vi "Keithley2200series_2.vi"() -> ()   [LabVIEW 2010]
uses:
  <vilib>/Utility/error.llb/whitespace.ctl
  C:/Users/rad/Desktop/Keithley 2200 Series Power Supplies Ver 1.2 (LV2009)/Keithley 2200 Series/Keithley 2200 Series.lvlib
panel:
  in  "ИС":string="5962-9683901MPA"
  in  "№ ИС":string
  out "SEE1 Count 2":dbl
  out "SEE1 Count":dbl
  in  "SEE th 2":dbl
  in  "SEE th 1":dbl
  in  "+ИП2":bool
  out "MEAS 2":string
  in  "Cml set 2":dbl
  in  "Function(0:Voltage) 3":u16(ring) items=["Voltage", "Current"]
  in  "Out set 2":dbl
  in  "VISA resource name 2":refnum<visa-resource-name>
  in  "Cml set":dbl
  in  "Function(0:Voltage) 2":u16(ring) items=["Voltage", "Current"]
  in  "Out set":dbl
  in  "Файл записи замеров":path
  out "MEAS":string
  in  "VISA resource name":refnum<visa-resource-name>
  in  "stop":bool
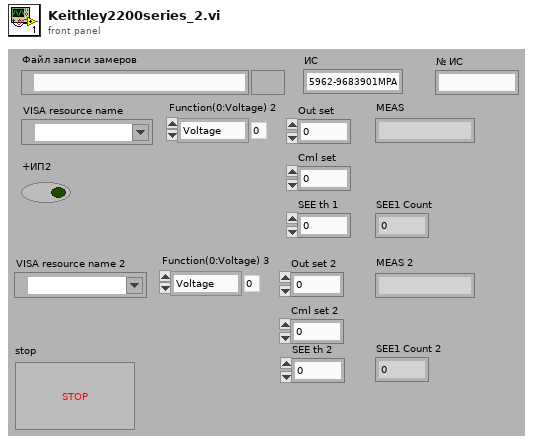
[diagram p1: front panel]
types:
  T1 = typedef "whitespace.ctl" = u16
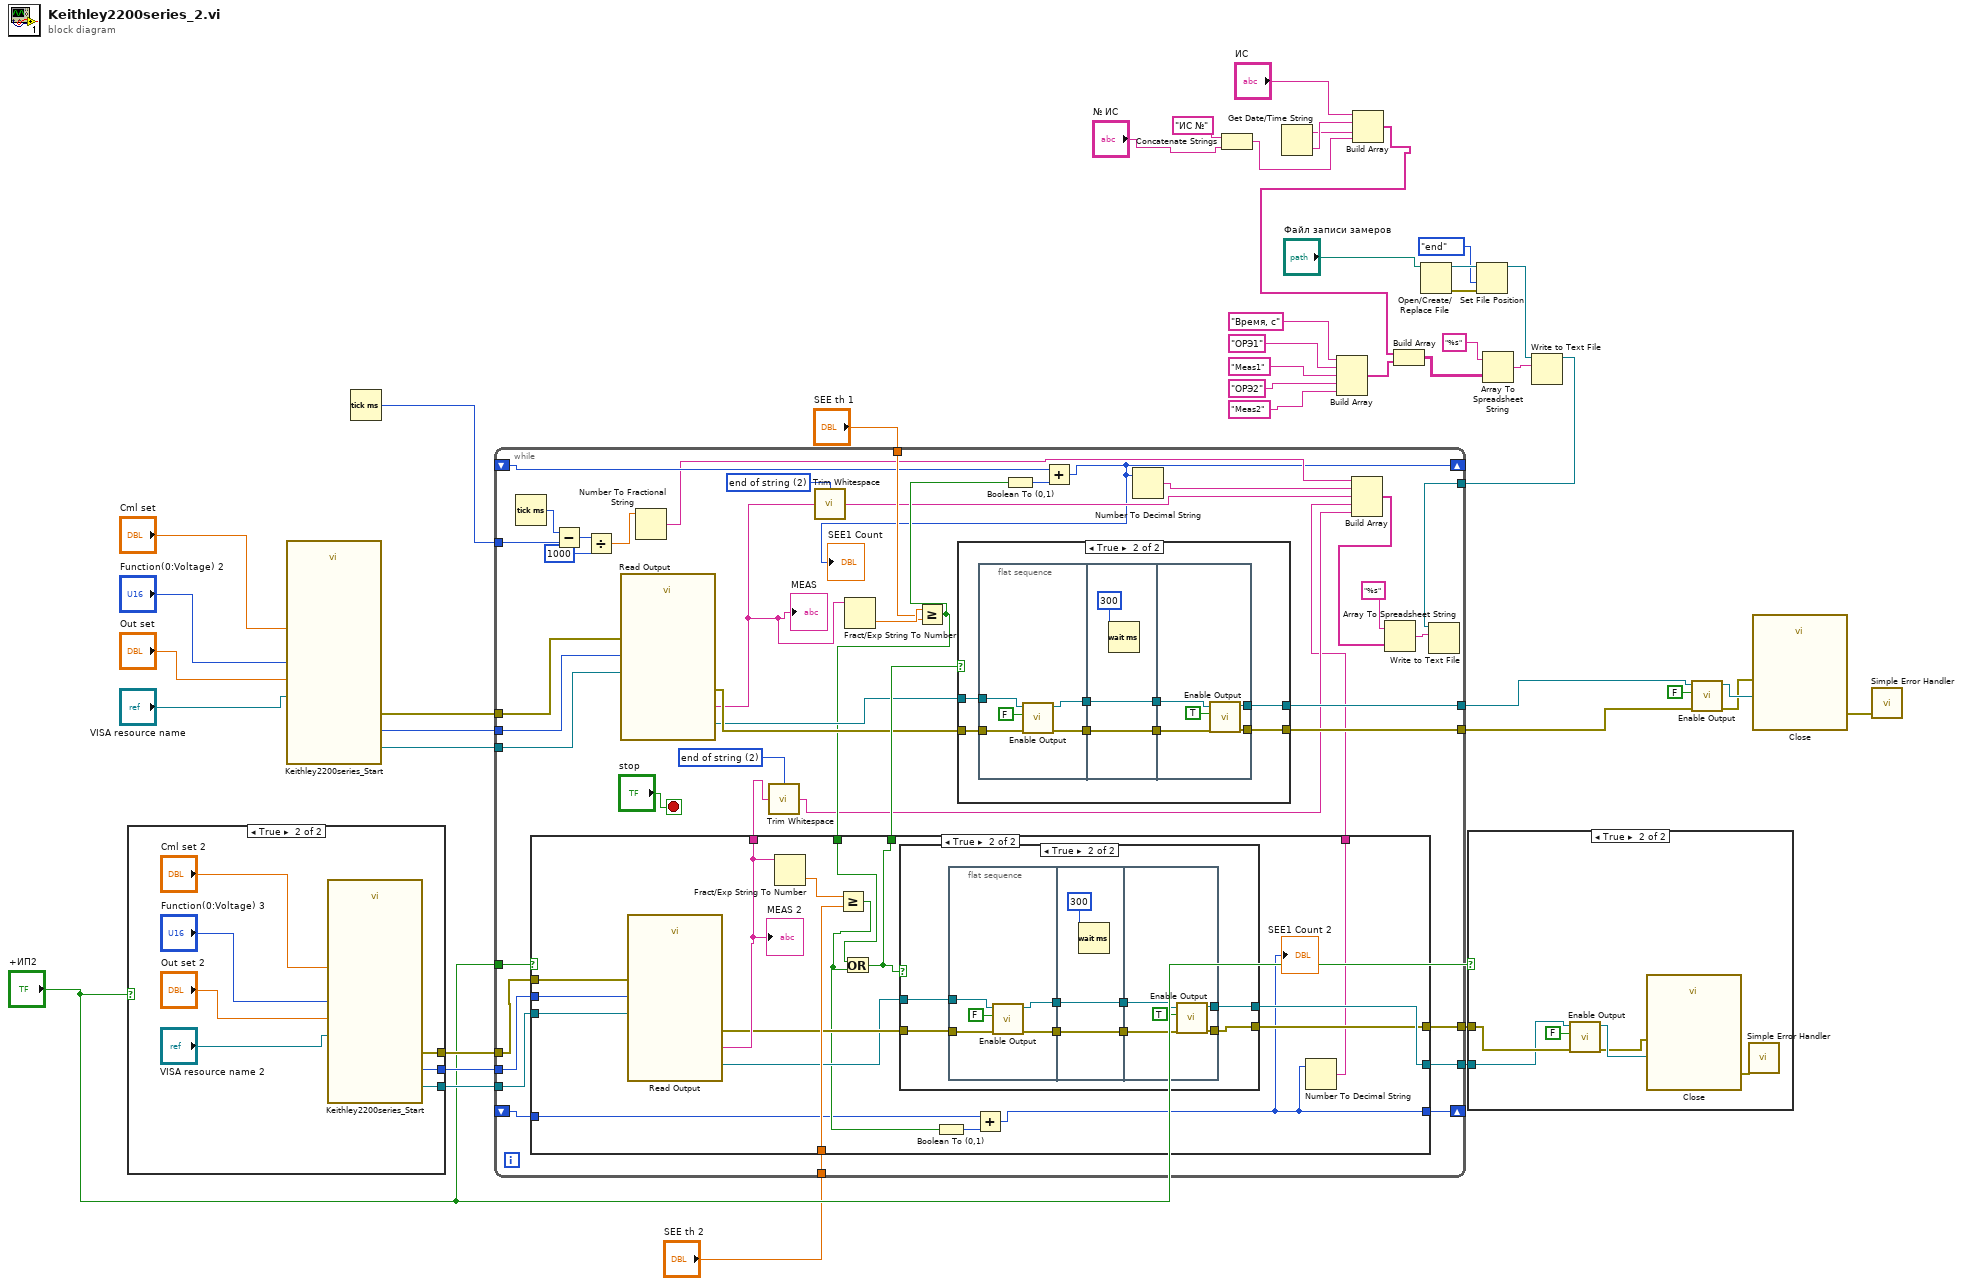
[diagram p0: block diagram]
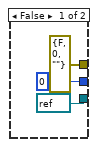
[diagram p3: hidden frame]
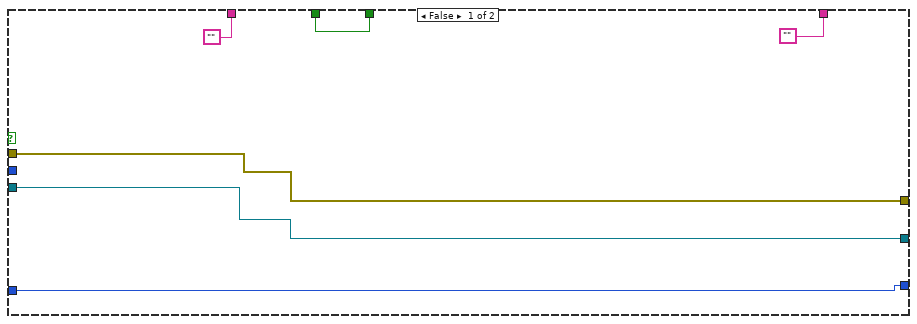
[diagram p5: hidden frame]
diagram:
  n1 = case shown="True" "+ИП2" {
    tunnel: [errorcluster {"status"=FALSE, "code"=0, "source"=""} ("error out 2") w50] -> w33
    tunnel: [0 ("Meas Func") w49] -> w32
    tunnel: [refnum<visa-resource-name> refnum ("VISA out") w48] -> w31
    frame False {
    }
    frame True {
      n2 = call "Keithley2200series_Start.vi"("VISA resource name 2"="VISA resource name 2", "Function(0:Voltage) 3"="Function(0:Voltage) 3", "Out set 2"="Out set 2", "Cml set 2"="Cml set 2") -> ("VISA out"=w48:refnum<visa-resource-name>, "Meas Func"=w49:i32, "error out 2"=w50:errorcluster)  [unwired: 1 in]
    }
  }
  n3 = call "Keithley2200series_Start.vi"("VISA resource name 2"="VISA resource name", "Function(0:Voltage) 3"="Function(0:Voltage) 2", "Out set 2"="Out set", "Cml set 2"="Cml set") -> ("VISA out"=w39:refnum<visa-resource-name>, "Meas Func"=w38:i32, "error out 2"=w37:errorcluster)  [unwired: 1 in]
  n4 = Tick Count (ms)() -> (millisecond timer value=w44:u32)
  n5 = Concatenate Strings("ИС №" ("string"), "№ ИС") -> (w5:string)
  n6 = Get Date/Time String() -> (date string=w8:string, time string=w9:string)  [unwired: 3 in]
  n7 = Build Array("Время, с", "ОРЭ1", "Meas1", "ОРЭ2", "Meas2") -> (w2:string[])
  n8 = Build Array("ИС", w9, w8, w5) -> (w1:string[])
  n9 = Build Array(w1, w2) -> (w3:string[][])
  n10 = Open/Create/Replace File(file path (use dialog)="Файл записи замеров") -> (refnum out=w13:refnum<file>, error out=w14:errorcluster)  [unwired: 5 in, 1 out]
  n11 = Set File Position(refnum=w13, from (0:start)=enum16{"start", "end", "current"}."end", error in=w14) -> (refnum out=w12:refnum<file>)  [unwired: 1 in, 1 out]
  n12 = Array To Spreadsheet String(array=w3, 3:"%s" ("format string")) -> (spreadsheet string=w17:string)  [unwired: 1 in]
  n13 = Write to Text File(file (use dialog)=w12, text=w17) -> (refnum out=w15:refnum<file>)  [unwired: 2 in, 2 out]
  n14 = while {
    tunnel: w44 -> [w95]
    tunnel: w39 -> [w91]
    tunnel: w38 -> [w90]
    tunnel: w37 -> [w89]
    tunnel: [w87] -> w35
    tunnel: [w86] -> w34
    tunnel: w33 -> [w85]
    tunnel: w32 -> [w84]
    tunnel: w31 -> [w83]
    tunnel: "+ИП2" -> [w82]
    tunnel: "SEE th 1" -> [w80]
    tunnel: "SEE th 2" -> [w79]
    tunnel: [w75] -> w24
    tunnel: [w74] -> w23
    shift-right: [w55] -> _
    shift-left: _ -> [w72]
    shift-right: [w69] -> _
    shift-left: _ -> [w70]
    tunnel: w15 -> [w66]
    stop <- "stop" stop-if-true
    w58 = T1 2 items=["both", "start of string", "end of string"] ("location (both)")
    w61 = T1 2 items=["both", "start of string", "end of string"] ("location (both)")
    n15 = Tick Count (ms)() -> (millisecond timer value=w96:u32)
    n16 = Subtract(x=w96, y=w95) -> (x-y=w94:u32)
    n17 = Divide(x=w94, y=u32 1000) -> (x/y=w92:dbl)
    n18 = call "Read Output.vi"("VISA resource name"=w91, "Measurement Function (0:Voltage)"=w90, "error in (no error)"=w89) -> ("VISA resource name out"=w76:refnum<visa-resource-name>, "Measurement"=w60:string, "error out"=w77:errorcluster)  [unwired: 10 in]
    "MEAS" <- w60
    n19 = Number To Fractional String(number=w92) -> (F-format string=w65:string)  [unwired: 3 in]
    n20 = call <vilib>:"Trim Whitespace.vi"("string"=w60, "location (both)"=w58) -> ("trimmed string"=w59:string)
    n21 = Fract/Exp String To Number(string=w60) -> (number=w81:dbl)  [unwired: 3 in, 1 out]
    n22 = Greater Or Equal?(x=w81, y=w80) -> (x >= y?=w71:bool)
    n23 = case shown="True" w82 {
      tunnel: [w125 w131] -> w87
      tunnel: [w124 w132] -> w86
      tunnel: ["" w139] -> w62
      tunnel: w85 -> [w125 w142]
      tunnel: w84 -> [_ w141]
      tunnel: w83 -> [w124 w140]
      tunnel: w79 -> [_ w138]
      tunnel: w71 -> [w123 w136]
      tunnel: [w123 w135] -> w78
      tunnel: w70 -> [w122 w128]
      tunnel: [w122 w126] -> w69
      tunnel: ["" w127] -> w56
      frame False {
      }
      frame True {
        n24 = call "Read Output.vi"("VISA resource name"=w140, "Measurement Function (0:Voltage)"=w141, "error in (no error)"=w142) -> ("VISA resource name out"=w133:refnum<visa-resource-name>, "Measurement"=w139:string, "error out"=w134:errorcluster)  [unwired: 10 in]
        "MEAS 2" <- w139
        n25 = Fract/Exp String To Number(string=w139) -> (number=w137:dbl)  [unwired: 3 in, 1 out]
        n26 = Greater Or Equal?(x=w137, y=w138) -> (x >= y?=w129:bool)
        n27 = Or(x=w136, y=w129) -> (x .or. y?=w135:bool)
        n28 = case shown="True" w135 {
          tunnel: w134 -> [w143 w148]
          tunnel: w133 -> [w144 w147]
          tunnel: [w144 w146] -> w132
          tunnel: [w143 w145] -> w131
          frame False {
          }
          frame True {
            n29 = flat-sequence {
              tunnel: w148 -> [w156]
              tunnel: w147 -> [w155]
              tunnel: [w154] -> w152
              tunnel: [w153] -> w151
              tunnel: [w159] -> w150
              tunnel: w152 -> [w159]
              tunnel: [w158] -> w149
              tunnel: w151 -> [w158]
              tunnel: w150 -> [w164]
              tunnel: w149 -> [w163]
              tunnel: [w162] -> w146
              tunnel: [w161] -> w145
              frame #0 {
                n30 = call "Enable Output.vi"("error in (no error)"=w156, "Enable Output (T: Enable)"=FALSE, "VISA resource name"=w155) -> ("error out"=w153:errorcluster, "VISA resource name out"=w154:refnum<visa-resource-name>)  [unwired: 7 in]
              }
              frame #1 {
                n31 = Wait (ms)(milliseconds to wait=u32 300) -> ()  [unwired: 1 out]
              }
              frame #2 {
                n32 = call "Enable Output.vi"("error in (no error)"=w163, "Enable Output (T: Enable)"=TRUE, "VISA resource name"=w164) -> ("error out"=w161:errorcluster, "VISA resource name out"=w162:refnum<visa-resource-name>)  [unwired: 7 in]
              }
            }
          }
        }
        n33 = Boolean To (0,1)(Boolean=w129) -> (0, 1=w130:i16)
        n34 = Add(x=w128, y=w130) -> (x+y=w126:i16)
        "SEE1 Count 2" <- w126
        n35 = Number To Decimal String(number=w126) -> (decimal integer string=w127:string)  [unwired: 1 in]
      }
    }
    n36 = call <vilib>:"Trim Whitespace.vi"("string"=w62, "location (both)"=w61) -> ("trimmed string"=w57:string)
    n37 = case shown="True" w78 {
      tunnel: w77 -> [w97 w106]
      tunnel: w76 -> [w98 w105]
      tunnel: [w98 w100] -> w75
      tunnel: [w97 w99] -> w74
      frame False {
      }
      frame True {
        n38 = flat-sequence {
          tunnel: w106 -> [w110]
          tunnel: w105 -> [w109]
          tunnel: [w108] -> w103
          tunnel: [w107] -> w101
          tunnel: [w113] -> w104
          tunnel: w103 -> [w113]
          tunnel: [w112] -> w102
          tunnel: w101 -> [w112]
          tunnel: w104 -> [w118]
          tunnel: w102 -> [w117]
          tunnel: [w116] -> w100
          tunnel: [w115] -> w99
          frame #0 {
            n39 = call "Enable Output.vi"("error in (no error)"=w110, "Enable Output (T: Enable)"=FALSE, "VISA resource name"=w109) -> ("error out"=w107:errorcluster, "VISA resource name out"=w108:refnum<visa-resource-name>)  [unwired: 7 in]
          }
          frame #1 {
            n40 = Wait (ms)(milliseconds to wait=u32 300) -> ()  [unwired: 1 out]
          }
          frame #2 {
            n41 = call "Enable Output.vi"("error in (no error)"=w117, "Enable Output (T: Enable)"=TRUE, "VISA resource name"=w118) -> ("error out"=w115:errorcluster, "VISA resource name out"=w116:refnum<visa-resource-name>)  [unwired: 7 in]
          }
        }
      }
    }
    n42 = Boolean To (0,1)(Boolean=w71) -> (0, 1=w73:i16)
    n43 = Add(x=w72, y=w73) -> (x+y=w55:i16)
    "SEE1 Count" <- w55
    n44 = Number To Decimal String(number=w55) -> (decimal integer string=w64:string)  [unwired: 1 in]
    n45 = Build Array(w65, w64, w59, w56, w57) -> (w63:string[])
    n46 = Array To Spreadsheet String(array=w63, 3:"%s" ("format string")) -> (spreadsheet string=w67:string)  [unwired: 1 in]
    n47 = Write to Text File(file (use dialog)=w66, text=w67) -> ()  [unwired: 2 in, 3 out]
  }
  n48 = case shown="True" "+ИП2" {
    tunnel: w35 -> [_ w169]
    tunnel: w34 -> [_ w168]
    frame False {
    }
    frame True {
      n49 = call "Enable Output.vi"("error in (no error)"=w169, "Enable Output (T: Enable)"=FALSE, "VISA resource name"=w168) -> ("error out"=w166:errorcluster, "VISA resource name out"=w167:refnum<visa-resource-name>)  [unwired: 7 in]
      n50 = call "Close.vi"("error in (no error)"=w166, "VISA resource name"=w167) -> ("error out"=w171:errorcluster)  [unwired: 9 in]
      n51 = call <vilib>:"Simple Error Handler.vi"("error in (no error)"=w171) -> ()  [unwired: 4 in, 5 out]
    }
  }
  n52 = call "Enable Output.vi"("error in (no error)"=w23, "Enable Output (T: Enable)"=FALSE, "VISA resource name"=w24) -> ("error out"=w28:errorcluster, "VISA resource name out"=w29:refnum<visa-resource-name>)  [unwired: 7 in]
  n53 = call "Close.vi"("error in (no error)"=w28, "VISA resource name"=w29) -> ("error out"=w36:errorcluster)  [unwired: 9 in]
  n54 = call <vilib>:"Simple Error Handler.vi"("error in (no error)"=w36) -> ()  [unwired: 4 in, 5 out]
